vi "ConnectK.vi"(1 "VISA resource name":refnum<visa-resource-name>, 2 "Baud rate":u32=9600, 5 "error in":errorcluster) -> (14 "Keyence":T2, 19 "error out":errorcluster)   [LabVIEW 2018]
uses:
  <vilib>/Instr/_visa.llb/VISA Flush IO Buffer Mask.ctl
  <vilib>/Instr/_visa.llb/VISA Configure Serial Port (Instr).vi
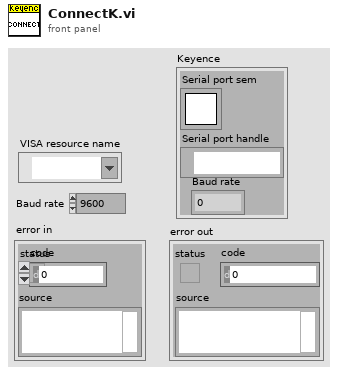
[diagram p1: front panel]
types:
  T1 = typedef "Semaphore RefNum" = refnum<k1>
  T2 = cluster{"Serial port sem":T1, "Serial port handle":refnum<visa-resource-name>, "Baud rate":u32}
  T3 = typedef "VISA Flush IO Buffer Mask.ctl" = u16
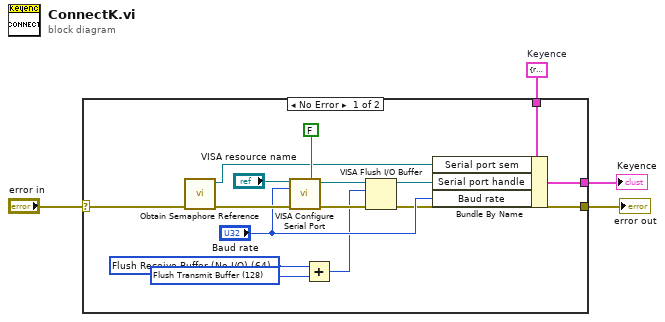
[diagram p0: block diagram]
diagram:
  w2 = T2 {"Serial port sem"=refnum, "Serial port handle"="", "Baud rate"=9600}  # Keyence
  n1 = case shown="No Error" "error in" {
    selector: "error in" -> [w17 w21]
    tunnel: [w10 w21] -> w3
    tunnel: [w14 w20] -> w1
    tunnel: w2 -> [w15 w20]
    frame No Error {
      w6 = T3 128 items=["Flush Receive Buffer"=16, "Write Transmit Buffer to Device"=32, "Flush Receive Buffer (No I/O)"=64, "Flush Transmit Buffer"=128] ("Mask")
      w7 = T3 64 items=["Flush Receive Buffer"=16, "Write Transmit Buffer to Device"=32, "Flush Receive Buffer (No I/O)"=64, "Flush Transmit Buffer"=128] ("Mask")
      n2 = call <vilib>:"Obtain Semaphore Reference.vi"("error in (no error)"=w17) -> ("error out"=w16:errorcluster, "semaphore"=w13:T1)  [unwired: 4 in, 1 out]
      n3 = call-poly "VISA Configure Serial Port"("VISA resource name"="VISA resource name", "Enable Termination\nChar (T)"=FALSE ("Enable Termination\nChar (T)"), "baud rate (9600)"="Baud rate", "error in (no error)"=w16) -> ("VISA resource name out"=w9:refnum<visa-resource-name>, "error out"=w11:errorcluster)  [unwired: 10 in]
      n4 = Add(x=w7, y=w6) -> (x+y=w5:T3)
      n5 = VISA Flush I/O Buffer(VISA resource name=w9, mask (16)=w5, error in (no error)=w11) -> (VISA resource name out=w8:refnum<visa-resource-name>, error out=w10:errorcluster)
      n6 = Bundle By Name(cluster=w15, "Serial port sem"=w13, "Serial port handle"=w8, "Baud rate"="Baud rate") -> (w14:T2)
    }
    frame Error {
    }
  }
  "error out" <- w3
  "Keyence" <- w1
